vi "Get Ini file sections.vi"(6 "error in (no error)":errorcluster, 9 "file (use dialog)":path) -> (0 "error out":errorcluster, 3 "Item names":string[](array[string]))   [LabVIEW 2013]
panel:
  in  "Items":u16(ring) items=["999999", "100016", "100013", "100005", "100010", "100063", "100041", "100042", "100062", "1001437", "100054", "100093", "100111", "100058", "100273", "100284", "100264", "100146", "100258", "100274", "100231", "100136", "100166", "100141", "100193", "100229", "end"]
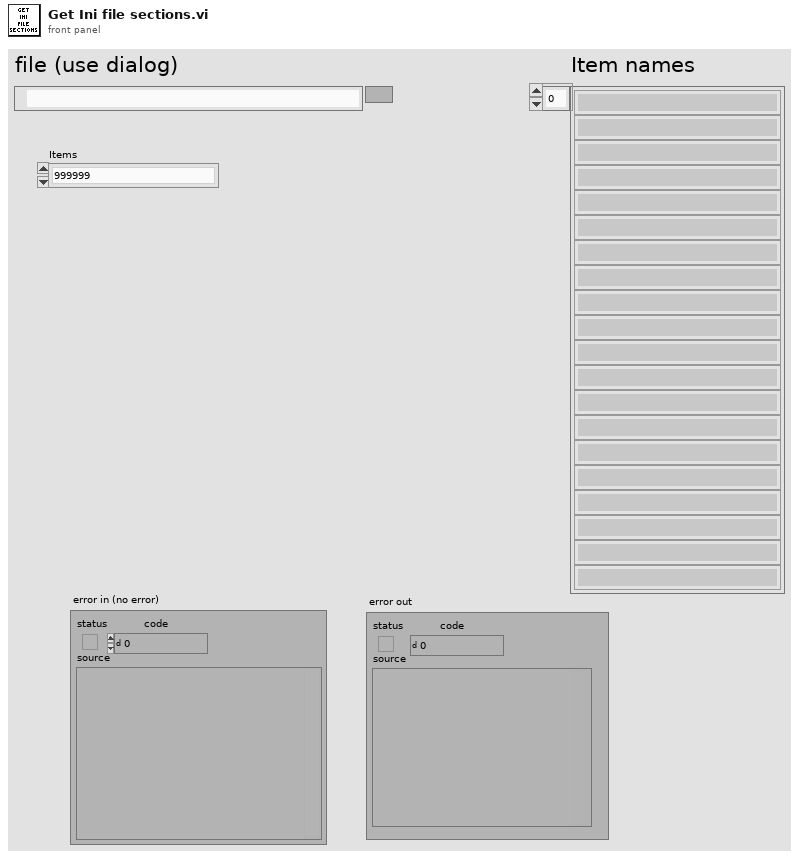
[diagram p1: front panel]
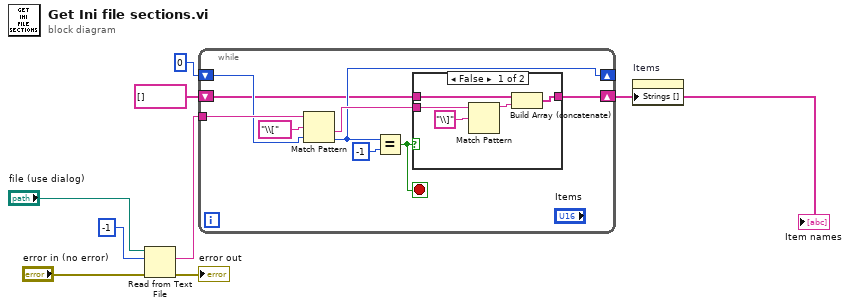
[diagram p0: block diagram]
diagram:
  n1 = Read from Text File(file (use dialog)="file (use dialog)", count=-1, error in="error in (no error)") -> (text=w5:string, error out=→"error out":errorcluster)  [unwired: 1 in, 2 out]
  n2 = while {
    tunnel: w5 -> [w17]
    shift-right: [w11] -> _
    shift-left: 0 -> [w12]
    shift-right: [w9] -> w1
    shift-left: string[] [] -> [w10]
    stop <- w14 stop-if-true
    n3 = Match Pattern(string=w17, regular expression="\\[", offset (0)=w12) -> (after substring=w13:string, offset past match=w11:i32)  [unwired: 2 out]
    n4 = Equal?(x=w11, y=-1) -> (x = y?=w14:bool)
    n5 = case shown="False" w14 {
      tunnel: w13 -> [w22 _]
      tunnel: w10 -> [w20 w23]
      tunnel: [w18 w23] -> w9
      frame False {
        n6 = Match Pattern(string=w22, regular expression="\\]") -> (before substring=w19:string)  [unwired: 1 in, 3 out]
        n7 = Build Array (concatenate)(w20, w19) -> (w18:string[])
      }
      frame True {
      }
    }
  }
  "Item names" <- w1
  n8 = property on="Items" class="Ring (strict)"("Strings []"=w1) -> ()  [unwired: 2 in, 2 out]
